vi "capturingSpectImage.vi"(8 "error in (no error)":errorcluster, 10 "command_captureSpectImage":T1, 11 "Model in":refnum<class "Model.lvclass">) -> (0 "error out":errorcluster, 3 "Model out":refnum<class "Model.lvclass">)   [LabVIEW 2016, in "Model.lvclass"]
uses:
  Model.lvclass
  ts_sallv_sedspectrometer/DataTypes/command_captureSpectImage.ctl
  Model.lvclass/Model.ctl
  <vilib>/express/express arith-compare/Formula/XNode/ExpressFormulaBlockNode.xnode
  ss_sedspectrometer/SEDSpectrometer/SEDSpectrometer.lvclass
  ts_sallv_sedspectrometer/SALLV_sedSpectrometer.lvlib
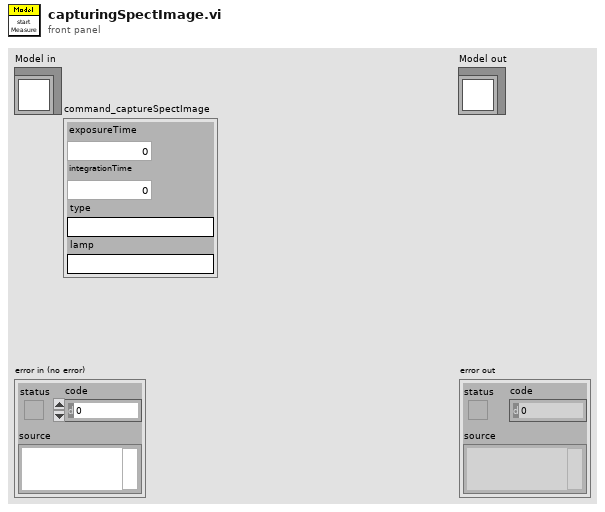
[diagram p1: front panel]
types:
  T1 = typedef "SALLV_sedSpectrometer.lvlib/command_captureSpectImage.ctl" = cluster{"exposureTime":sgl, "integrationTime":sgl, "type":string, "lamp":string}
  T2 = cluster{"StartPixel":u16, "StopPixel":u16, "IntegrationTime":sgl, "IntegrationDelay":u32, "NrAverages":u32, "DarkCorrectionType":cluster{"Enable CorDynDark":u8, "ForgetPercentage":u8}, "SmoothingType":cluster{"SmoothPix":u16, "SmoothModel":u8}, "SatDetection":u8, "TriggerType":cluster{"Trigger Mode":u8, "Trigger Source":u8, "Trigger SourceType":u8}, "ControlSettingsType":cluster{"StrobeControl":u16, "LaserDelay":u32, "LaserWidth":u32, "LaserWaveLength":sgl, "StoreToRam":u16}}
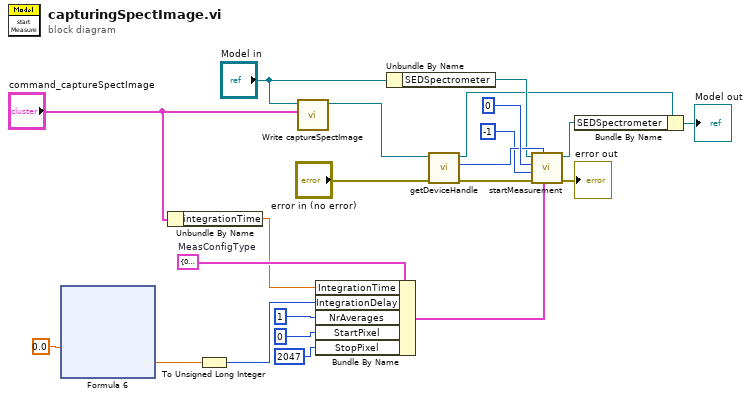
[diagram p0: block diagram]
diagram:
  w22 = T2 {"StartPixel"=0, "StopPixel"=0, "IntegrationTime"=0.0, "IntegrationDelay"=0, "NrAverages"=0, "DarkCorrectionType"={"Enable CorDynDark"=0, "ForgetPercentage"=0}, "SmoothingType"={"SmoothPix"=0, "SmoothModel"=0}, "SatDetection"=0, "TriggerType"={"Trigger Mode"=0, "Trigger Source"=0, "Trigger SourceType"=0}, "ControlSettingsType"={"StrobeControl"=0, "LaserDelay"=0, "LaserWidth"=0, "LaserWaveLength"=0.0, "StoreToRam"=0}}  # MeasConfigType
  n1 = xnode "Formula 6"("X1"=0.0) -> ("Result"=w20:dbl)  [unwired: 1 in, 1 out]
  n2 = Unbundle By Name("command_captureSpectImage") -> ("integrationTime"=w21:sgl)
  n3 = To Unsigned Long Integer(number=w20) -> (unsigned 32bit integer=w19:u32)
  n4 = call-dynamic "Write captureSpectImage.vi"("command_captureSpectImage"="command_captureSpectImage", "Model in"="Model in") -> ("Model out"=w1:refnum<class "Model.lvclass">)  [unwired: 8 in, 1 out]
  n5 = Bundle By Name(cluster=w22, "IntegrationTime"=w21, "IntegrationDelay"=w19, "NrAverages"=u32 1, "StartPixel"=u16 0, "StopPixel"=u16 2047) -> (w16:T2)
  n6 = Unbundle By Name("Model in") -> ("SEDSpectrometer"=w11:refnum<class "SEDSpectrometer.lvclass">)
  n7 = call-dynamic "getDeviceHandle.vi"("error in (no error)"="error in (no error)", "Model in"=w1) -> ("error out"=w12:errorcluster, "Device"=w14:i32, "Model out"=w10:refnum<class "Model.lvclass">)  [unwired: 7 in]
  n8 = call "startMeasurement.vi"("MeasConfigType"=w16, "Device Handle"=w14, "error in (no error)"=w12, "NumOfScans"=i16 -1, "a_hWnd"=0, "SEDSpectrometer in"=w11) -> ("error out"=→"error out":errorcluster, "SEDSpectrometer out"=w8:refnum<class "SEDSpectrometer.lvclass">)  [unwired: 2 in, 2 out]
  n9 = Bundle By Name(cluster=w10, "SEDSpectrometer"=w8) -> (→"Model out":refnum<class "Model.lvclass">)
